vi "simple_test.vi"(1 "Arr Refnum":refnum<vi>) -> ()   [LabVIEW 2010]
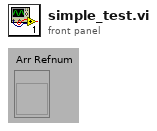
[diagram p1: front panel]
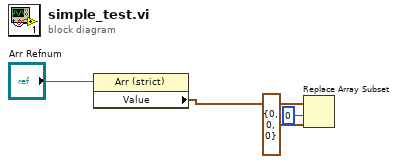
[diagram p0: block diagram]
diagram:
  n1 = property class="Arr (strict)"(reference="Arr Refnum") -> ("Value"=w3:cluster{"MSG":i16, "Param":i32, "type":i16}[])  [unwired: 1 in, 2 out]
  n2 = Replace Array Subset(array=w3, new element=cluster{"MSG":i16, "Param":i32, "type":i16} {"MSG"=0, "Param"=0, "type"=0} ("new element/subarray"), index=0) -> ()  [unwired: 1 out]
